vi "FMV - get header (mclb).vi"(8 "error in (no error)":errorcluster, 11 "JSON string":string) -> (0 "error out":errorcluster, 3 "value":string)   [LabVIEW 2020, in "ui-testing.lvlib"]
doc: "copyright: Thomas Zilliox©"
uses:
  ui-testing.lvlib
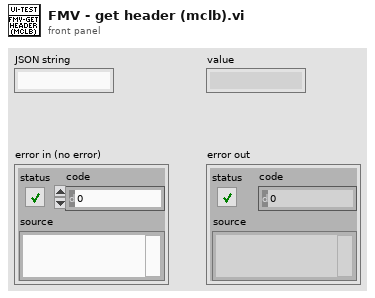
[diagram p1: front panel]
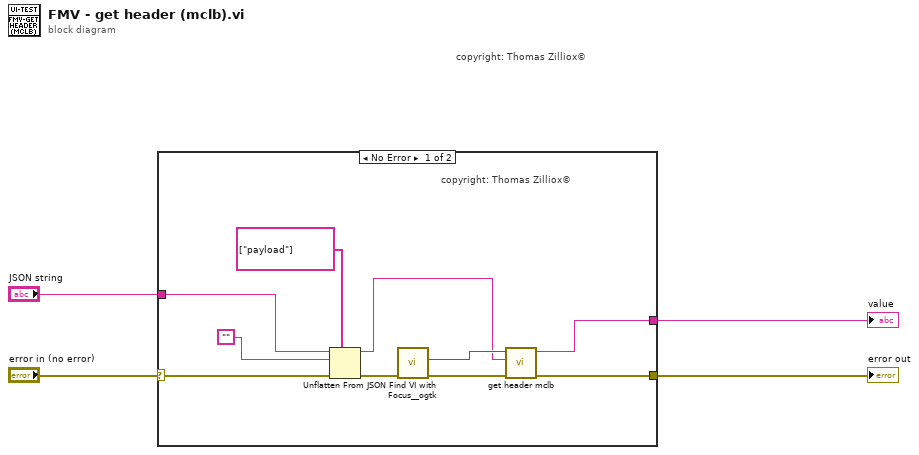
[diagram p0: block diagram]
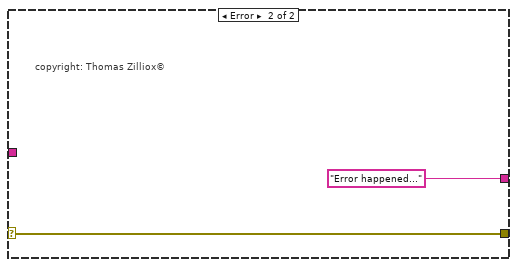
[diagram p2: hidden frame]
diagram:
  # "copyright: Thomas Zilliox©"
  n1 = case shown="No Error" "error in (no error)" {
    selector: "error in (no error)" -> [w10 w16]
    tunnel: "JSON string" -> [w11 _]
    tunnel: [w5 w16] -> w3
    tunnel: [w7 "Error happened..."] -> w2
    frame No Error {
      # "copyright: Thomas Zilliox©"
      n2 = Unflatten From JSON(path=string[] ["payload"], JSON string=w11, type and defaults="", error in (no error)=w10) -> (value=w8:string, error out=w13:errorcluster)  [unwired: 3 in]
      n3 = call <userlib>:"Find VI with Focus__ogtk.vi"("error in"=w13) -> ("error out"=w6:errorcluster, "VI with Focus"=w9:refnum<vi>)  [unwired: 6 in, 3 out]
      n4 = call "get header mclb.vi"("error in (no error)"=w6, "Control label"=w8, "VI (Caller)"=w9) -> ("error out"=w5:errorcluster, "headers"=w7:string)  [unwired: 7 in]
    }
    frame Error {
      # "copyright: Thomas Zilliox©"
    }
  }
  "error out" <- w3
  "value" <- w2
